vi "Write Completion Notification Msg.vi"(8 "error in (no error)":errorcluster, 10 "Async Methods Actor.lvlib:Completion Ack Msg.lvclass":refnum<class "Completion Notification Msg.lvclass">, 11 "Async Message in":refnum<class "Async Message.lvclass">) -> (0 "error out":errorcluster, 3 "Async Message out":refnum<class "Async Message.lvclass">)   [LabVIEW 2021, in "Async Methods Actor.lvlib" / "Async Message.lvclass"]
doc: "Sets a concrete subclass of the \"Completion Notification Msg.lvclass\" abstract message to notify the caller (specified by the \"Caller Enqueuer\" property) about completion of Async Message. The caller will receive the completed Async Message allowing the access by means of it property to its GUID and FQN as well as the remaining number of \"Call and Collect\" Async Messages of the same type. To enable the callee Async Methods Acor to notify completion both this property and the \"Caller Enqueuer\" must be properly set."
uses:
  Async Message.lvclass
  Completion Notification Msg/Completion Notification Msg.lvclass
  Async Message.lvclass/Async Message.ctl
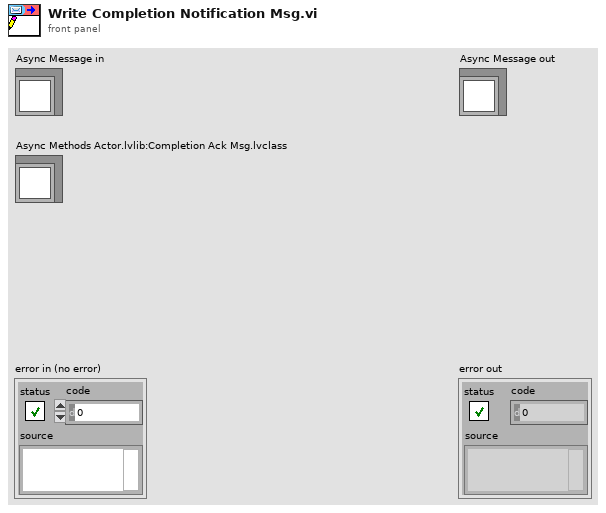
[diagram p1: front panel]
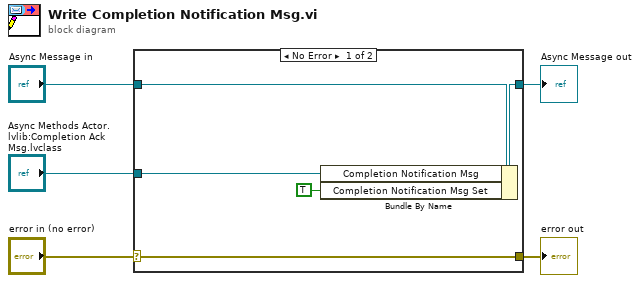
[diagram p0: block diagram]
diagram:
  n1 = case shown="No Error" "error in (no error)" {
    selector: "error in (no error)" -> [w10 w11]
    tunnel: [w10 w11] -> w4
    tunnel: [w8 w12] -> w2
    tunnel: "Async Message in" -> [w9 w12]
    tunnel: "Async Methods Actor.lvlib:Completion Ack Msg.lvclass" -> [w7 _]
    frame No Error {
      n2 = Bundle By Name(cluster=w9, "Completion Notification Msg"=w7, "Completion Notification Msg Set"=TRUE) -> (w8:refnum<class "Async Message.lvclass">)
    }
    frame Error {
    }
  }
  "error out" <- w4
  "Async Message out" <- w2
